vi "R5pHControl_Status.vi"(7 "LabVIEW Web Service Request":refnum<class "Web Request.lvclass">) -> ()   [LabVIEW 2016]
uses:
  <vilib>/wsapi/Web Request.lvclass
  R5Controls/R5pH_Status.ctl
  Controls/pH_Manual Standard.ctl
  Controls/pH_SetParams Standard.ctl
panel:
  out "pH Data":T1
  # "Use the Web Service Request input terminal to call the VIs on the Web Services palette. Do not remove it from the connector pane unless you don't need access to the palette."
  # "Each additional control wired to the connector pane will be available as an input in the URL. To include an indicator in terminal-mode output (the default setting), it must also be wired to the connector pane."
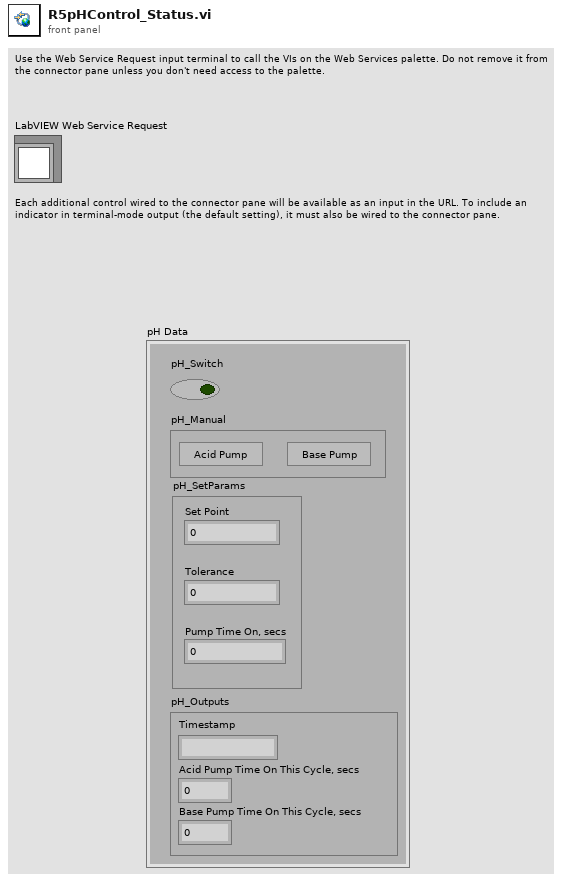
[diagram p1: front panel]
types:
  T1 = typedef "R5pH_Status.ctl" = cluster{"pH_Switch":bool, "pH_Manual":T2, "pH_SetParams":T3, "pH_Outputs":cluster{"Timestamp":string, "Acid Pump Time On This Cycle, secs":dbl, "Base Pump Time On This Cycle, secs":dbl}}
  T2 = typedef "pH_Manual Standard.ctl" = cluster{"Acid Pump":bool, "Base Pump":bool}
  T3 = typedef "pH_SetParams Standard.ctl" = cluster{"Set Point":dbl, "Tolerance":dbl, "Pump Time On, secs":dbl}
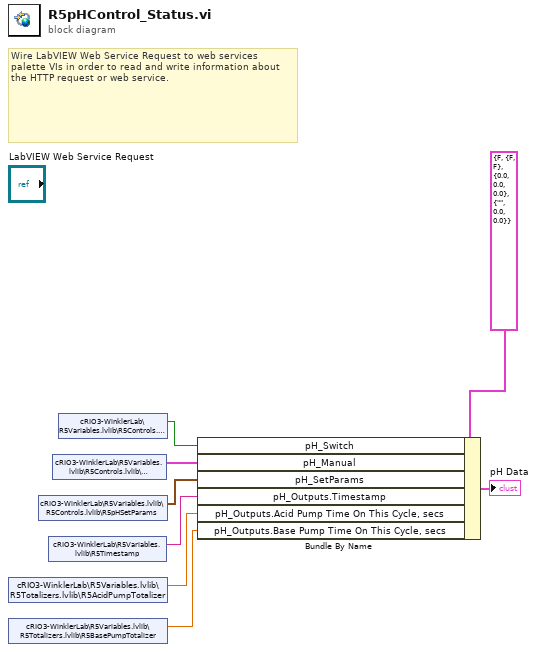
[diagram p0: block diagram]
diagram:
  # "Wire LabVIEW Web Service Request to web services palette VIs in order to read and write information about the HTTP request or web service."
  n1 = shared-variable "cRIO3-WinklerLab\\R5Variables.lvlib\\R5Totalizers.lvlib\\R5AcidPumpTotalizer"() -> (w7:dbl)  [unwired: 1 in, 1 out]
  n2 = shared-variable "cRIO3-WinklerLab\\R5Variables.lvlib\\R5Totalizers.lvlib\\R5BasePumpTotalizer"() -> (w8:dbl)  [unwired: 1 in, 1 out]
  n3 = shared-variable "cRIO3-WinklerLab\\R5Variables.lvlib\\R5Controls.lvlib\\R5pHSetParams"() -> (w5:T3)  [unwired: 1 in, 1 out]
  n4 = shared-variable "cRIO3-WinklerLab\\R5Variables.lvlib\\R5Timestamp"() -> (w6:string)  [unwired: 1 in, 1 out]
  n5 = shared-variable "cRIO3-WinklerLab\\R5Variables.lvlib\\R5Controls.lvlib\\R5pHManual"() -> (w4:cluster{"Acid Pump":bool, "Base Pump":bool})  [unwired: 1 in, 1 out]
  n6 = shared-variable "cRIO3-WinklerLab\\R5Variables.lvlib\\R5Controls.lvlib\\R5pHSwitch"() -> (w3:bool)  [unwired: 1 in, 1 out]
  n7 = Bundle By Name(cluster=T1 {"pH_Switch"=FALSE, "pH_Manual"={"Acid Pump"=FALSE, "Base Pump"=FALSE}, "pH_SetParams"={"Set Point"=0.0, "Tolerance"=0.0, "Pump Time On, secs"=0.0}, "pH_Outputs"={"Timestamp"="", "Acid Pump Time On This Cycle, secs"=0.0, "Base Pump Time On This Cycle, secs"=0.0}} ("pHData"), "pH_Switch"=w3, "pH_Manual"=w4, "pH_SetParams"=w5, "pH_Outputs.Timestamp"=w6, "pH_Outputs.Acid Pump Time On This Cycle, secs"=w7, "pH_Outputs.Base Pump Time On This Cycle, secs"=w8) -> (→"pH Data":T1)
